vi "split_channels_syncAftercnt.vi"(0 "stamps":i64[](array[numeric]), 1 "last_sync_num_in":i32, 5 "channels":u32[](array[numeric]), 9 "sync_channel":u32, 11 "error constant":errorcluster, 12 "syncAfter":bool) -> (3 "last_sync_num_out":i32, 4 "count_channels":u32[](array[numeric]), 6 "n_sync":i32[](array[numeric]), 8 "time_delays":i64[](array[numeric]), 10 "leftovers":i64[](array[numeric]), 14 "leftover_channels":i32[](array[numeric]), 15 "error IO":errorcluster)   [LabVIEW 2018]
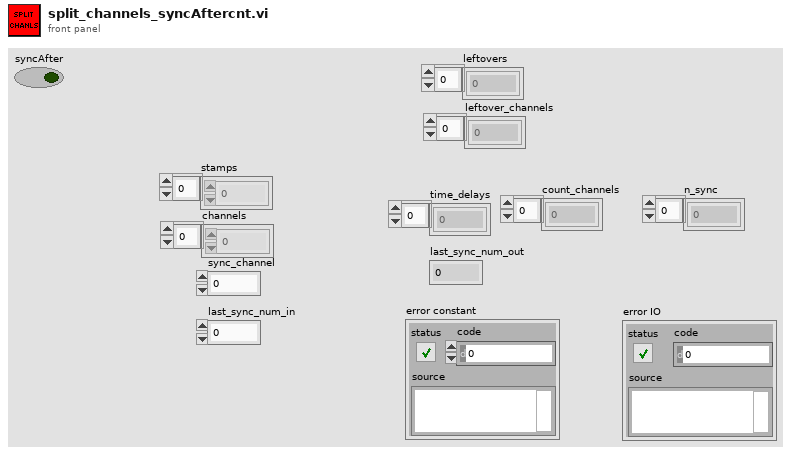
[diagram p1: front panel]
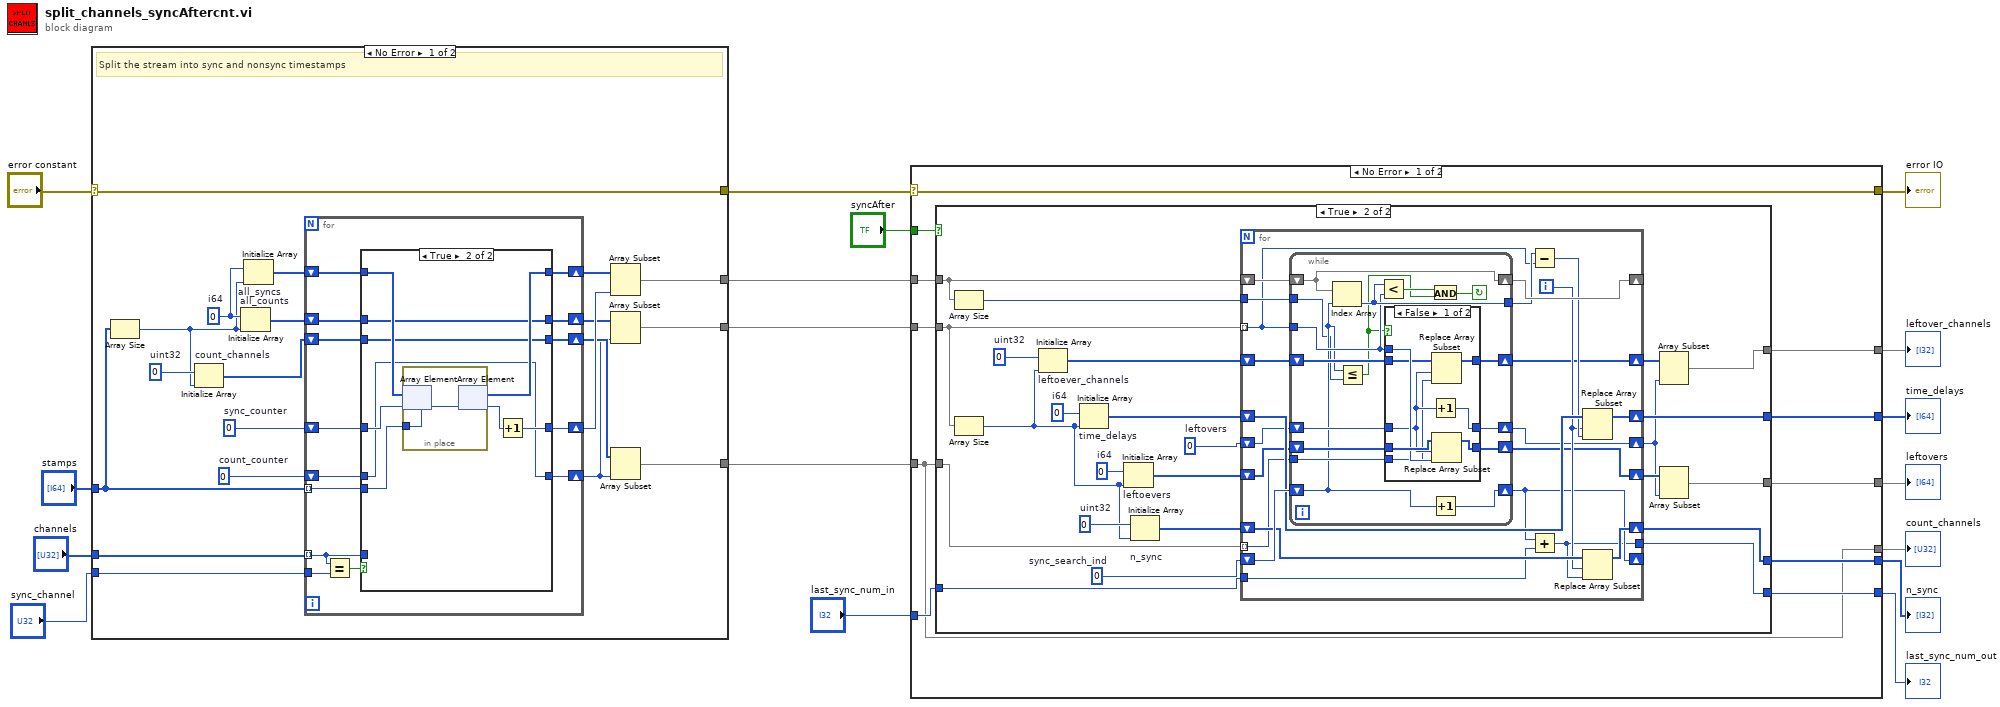
[diagram p0: block diagram]
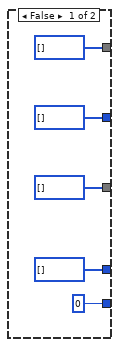
[diagram p2: hidden frame]
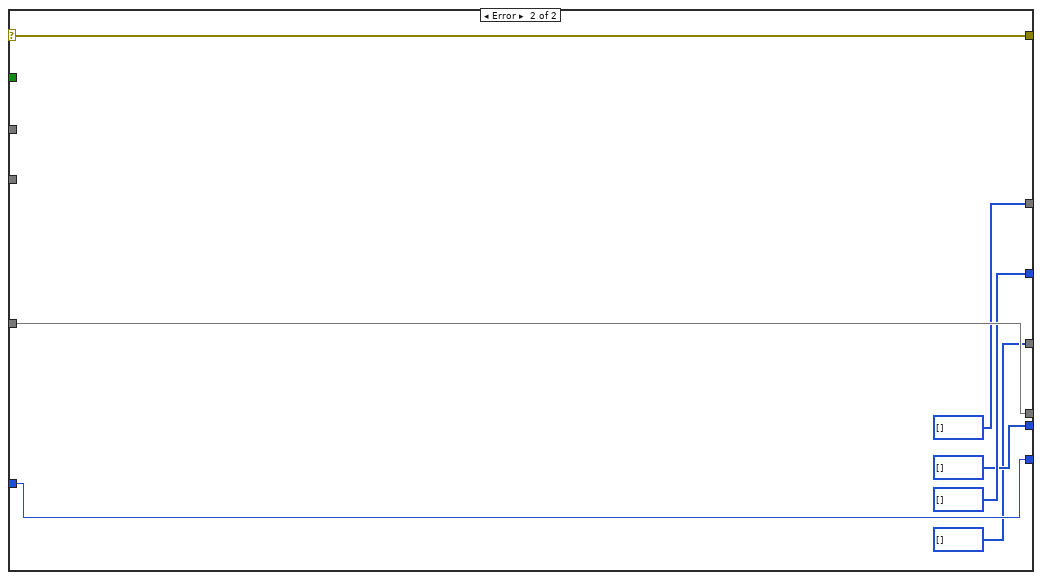
[diagram p4: hidden frame]
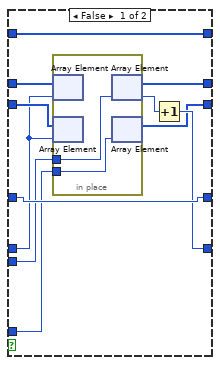
[diagram p5: hidden frame]
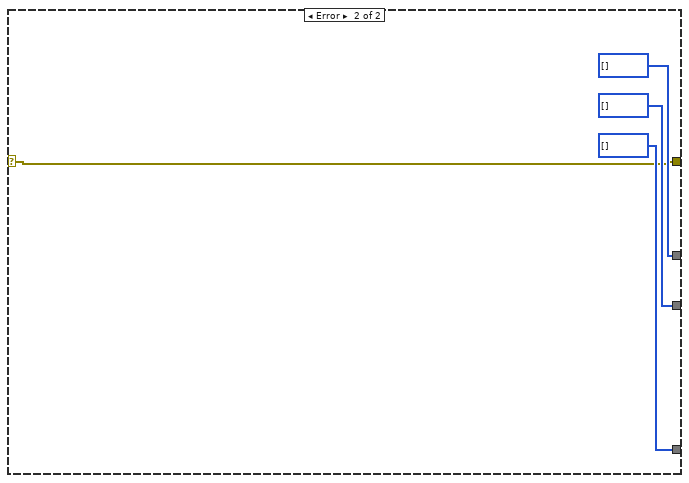
[diagram p6: hidden frame]
diagram:
  n1 = case shown="No Error" "error constant" {
    selector: "error constant" -> [w26 w75]
    tunnel: "channels" -> [w37 _]
    tunnel: "sync_channel" -> [w31 _]
    tunnel: "stamps" -> [w28 _]
    tunnel: [w26 w75] -> w13
    tunnel: [w23 i64[] []] -> w11
    tunnel: [w21 i64[] []] -> w12
    tunnel: [w18 u32[] []] -> w10
    frame No Error {
      w34 = 0  # count_counter
      w33 = 0  # sync_counter
      w29 = u32 0  # uint32
      w30 = i64 0  # i64
      # "Split the stream into sync and nonsync timestamps"
      n2 = Array Size(array=w28) -> (size(s)=w27:i32)
      n3 = Initialize Array "count_channels"(w29, w27) -> (w36:u32[])
      n4 = Initialize Array "all_counts"(w30, w27) -> (w35:i64[])
      n5 = Initialize Array "all_syncs"(w30, w27) -> (w32:i64[])
      n6 = for {
        tunnel: w28 -> [w38] mode=indexing
        tunnel: w31 -> [w51]
        shift-right: [w46] -> w25
        shift-left: w32 -> [w49]
        shift-right: [w47] -> w24
        shift-left: w33 -> [w48]
        shift-right: [w43] -> w19
        shift-left: w34 -> [w45]
        shift-right: [w42] -> w22
        shift-left: w35 -> [w44]
        shift-right: [w40] -> w20
        shift-left: w36 -> [w41]
        tunnel: w37 -> [w39] mode=indexing
        n7 = Equal?(x=w39, y=w51) -> (x = y?=w50:bool)
        n8 = case shown="True" w50 {
          tunnel: w49 -> [w62 w73]
          tunnel: w48 -> [w61 w72]
          tunnel: [w61 w70] -> w47
          tunnel: w39 -> [w52 _]
          tunnel: [w62 w69] -> w46
          tunnel: w45 -> [w55 w67]
          tunnel: w44 -> [w60 w68]
          tunnel: [w58 w67] -> w43
          tunnel: [w57 w68] -> w42
          tunnel: w41 -> [w56 w66]
          tunnel: [w54 w66] -> w40
          tunnel: w38 -> [w53 w65]
          frame False {
            n9 = in-place {
              in-place-border: w53 -> [w64]
              in-place-border: w52 -> [w63]
              n10 = in-place-array #1(w60, w55) -> ()  [unwired: 1 out]
              n11 = in-place-array #2(w56, w55) -> ()  [unwired: 1 out]
              n12 = in-place-array #1(w64) -> (w57:i64[], w59:i32)
              n13 = in-place-array #2(w63) -> (w54:u32[])  [unwired: 1 out]
            }
            n14 = Increment(x=w59) -> (x+1=w58:i32)
          }
          frame True {
            n15 = in-place {
              in-place-border: w65 -> [w74]
              n16 = in-place-array #3(w73, w72) -> ()  [unwired: 1 out]
              n17 = in-place-array #3(w74) -> (w69:i64[], w71:i32)
            }
            n18 = Increment(x=w71) -> (x+1=w70:i32)
          }
        }
      }
      n19 = Array Subset(array=w25, length=w24) -> (w23:i64[])  [unwired: 1 in]
      n20 = Array Subset(array=w22, length=w19) -> (w21:i64[])  [unwired: 1 in]
      n21 = Array Subset(array=w20, length=w19) -> (w18:u32[])  [unwired: 1 in]
    }
    frame Error {
    }
  }
  n22 = case shown="No Error" w13 {
    selector: w13 -> [w83 w170]
    tunnel: w12 -> [w89 _]
    tunnel: w11 -> [w88 _]
    tunnel: w10 -> [w80 w174]
    tunnel: [w80 w174] -> w9
    tunnel: [w87 i64[] []] -> w8
    tunnel: [w86 i32[] []] -> w7
    tunnel: "last_sync_num_in" -> [w85 w171]
    tunnel: [w84 w171] -> w5
    tunnel: [w83 w170] -> w4
    tunnel: "syncAfter" -> [w82 _]
    tunnel: [w81 i64[] []] -> w2
    tunnel: [w79 i32[] []] -> w1
    frame No Error {
      n23 = case shown="True" w82 {
        tunnel: w89 -> [_ w116]
        tunnel: w88 -> [_ w113]
        tunnel: [i64[] [] w111] -> w87
        tunnel: [i32[] [] w109] -> w86
        tunnel: w85 -> [_ w108]
        tunnel: [0 w107] -> w84
        tunnel: [i64[] [] w102] -> w81
        tunnel: w80 -> [_ w98]
        tunnel: [i32[] [] w95] -> w79
        frame False {
        }
        frame True {
          w101 = 0  # uint32
          w104 = 0  # leftovers
          w106 = i64 0  # i64
          w115 = 0  # sync_search_ind
          w117 = 0  # uint32
          w118 = i64 0  # i64
          n24 = Array Size(array=w113) -> (size(s)=w112:i32)
          n25 = Array Size(array=w116) -> (size(s)=w100:i32)
          n26 = Initialize Array "leftoever_channels"(w101, w100) -> (w99:i32[])
          n27 = Initialize Array "time_delays"(w118, w100) -> (w114:i64[])
          n28 = Initialize Array "leftoevers"(w106, w100) -> (w105:i64[])
          n29 = Initialize Array "n_sync"(w117, w100) -> (w110:i32[])
          n30 = for {
            tunnel: w116 -> [w133] mode=indexing
            shift-right: [w137] -> _
            shift-left: w113 -> [w140]
            shift-right: [w135] -> w111
            shift-left: w114 -> [w136]
            shift-right: [w128] -> _
            shift-left: w115 -> [w139]
            tunnel: w112 -> [w138]
            shift-right: [w129] -> w109
            shift-left: w110 -> [w131]
            tunnel: w108 -> [w127]
            tunnel: [w126] -> w107
            shift-right: [w123] -> w103
            shift-left: w105 -> [w125]
            shift-right: [w122] -> w96
            shift-left: w104 -> [w124]
            shift-right: [w119] -> w97
            shift-left: w99 -> [w121]
            tunnel: w98 -> [w120] mode=indexing
            i -> [w130]
            n31 = while {
              shift-right: [w153] -> w137
              shift-left: w140 -> [w153]
              shift-right: [w156] -> w128
              shift-left: w139 -> [w143]
              tunnel: w133 -> [w149]
              tunnel: w138 -> [w142]
              tunnel: [w152] -> w134
              shift-right: [w148] -> w123
              shift-left: w125 -> [w151]
              shift-right: [w147] -> w122
              shift-left: w124 -> [w150]
              tunnel: w120 -> [w145]
              shift-right: [w144] -> w119
              shift-left: w121 -> [w146]
              stop <- w154 continue-if-true
              n32 = Index Array(array=w153, index=w143) -> (element=w152:i64)
              n33 = Less Or Equal?(x=w143, y=w142) -> (x <= y?=w141:bool)
              n34 = Less?(x=w152, y=w149) -> (x < y?=w155:bool)
              n35 = case shown="False" w141 {
                tunnel: w151 -> [w164 w167]
                tunnel: w150 -> [w159 w166]
                tunnel: w149 -> [w163 _]
                tunnel: [w162 w167] -> w148
                tunnel: [w161 w166] -> w147
                tunnel: w146 -> [w160 w165]
                tunnel: w145 -> [w158 _]
                tunnel: [w157 w165] -> w144
                frame False {
                  n36 = Increment(x=w159) -> (x+1=w161:i32)
                  n37 = Replace Array Subset(array=w160, new element=w158, index=w159) -> (w157:i32[])
                  n38 = Replace Array Subset(array=w164, new element=w163, index=w159) -> (w162:i64[])
                }
                frame True {
                }
              }
              n39 = And(x=w155, y=w141) -> (x .and. y?=w154:bool)
              n40 = Increment(x=w143) -> (x+1=w156:i32)
            }
            n41 = Subtract(x=w134, y=w133) -> (x-y=w132:i64)
            n42 = Add(x=w128, y=w127) -> (x+y=w126:i32)
            n43 = Replace Array Subset(array=w136, new element=w132, index=w130) -> (w135:i64[])
            n44 = Replace Array Subset(array=w131, new element=w126, index=w130) -> (w129:i32[])
          }
          n45 = Array Subset(array=w97, length=w96) -> (w95:i32[])  [unwired: 1 in]
          n46 = Array Subset(array=w103, length=w96) -> (w102:i64[])  [unwired: 1 in]
        }
      }
    }
    frame Error {
    }
  }
  "count_channels" <- w9
  "time_delays" <- w8
  "n_sync" <- w7
  "last_sync_num_out" <- w5
  "error IO" <- w4
  "leftovers" <- w2
  "leftover_channels" <- w1
